vi "Initialise.vi"(8 "error in (no error)":errorcluster, 10 "Window Height":i32=480, 11 "Window Width":i32=640) -> (0 "error out":errorcluster, 3 "Renderer out":refnum<class "Renderer.lvclass">)   [LabVIEW 2021, in "Renderer.lvclass"]
uses:
  Renderer.lvclass
  Renderer.lvclass/Renderer.ctl
  LabSDL2/Source/Libraries/LibSDL2 Wrapper/LibSDL2.lvlib
  LabSDL2/Source/Libraries/LibSDL2_Image Wrapper/LibSDL2_Image.lvlib
  LabSDL2/Source/Libraries/LibSDL2_TTF Wrapper/LibSDL2_TTF.lvlib
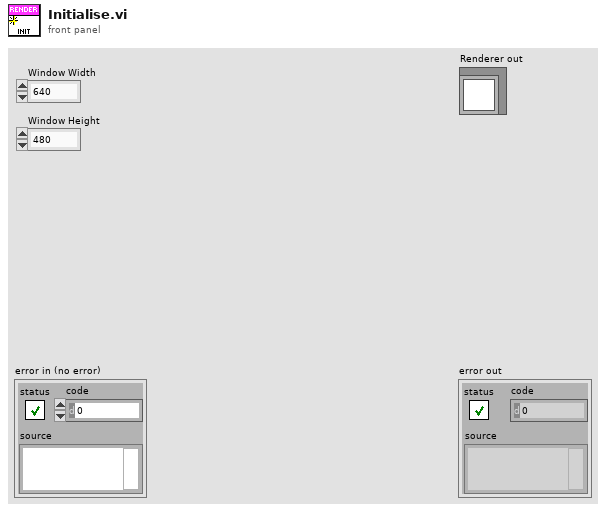
[diagram p1: front panel]
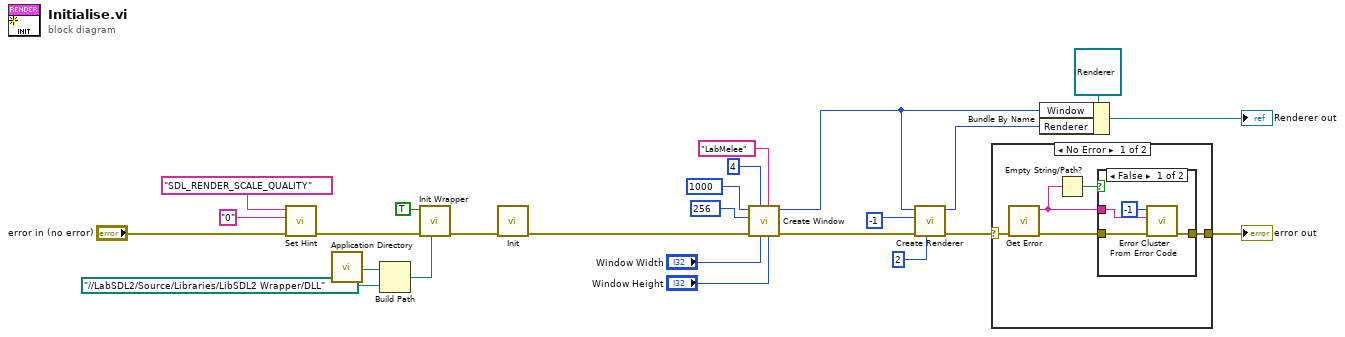
[diagram p0: block diagram]
diagram:
  n1 = call "Set Hint.vi"("error in"="error in (no error)", "Value"="0", "Name"="SDL_RENDER_SCALE_QUALITY") -> ("error out"=w22:errorcluster)  [unwired: 7 in, 1 out]
  n2 = call <vilib>:"Application Directory.vi"() -> ("Application Directory"=w14:path)
  n3 = Build Path(base path=w14, name or relative path=path "../../LabSDL2/Source/Libraries/LibSDL2 Wrapper/DLL" ("DLL Directory")) -> (appended path=w12:path)
  n4 = call "Init Wrapper.vi"("DLL Directory"=w12, "error in"=w22, "PNG (F)"=TRUE ("PNG")) -> ("error out"=w11:errorcluster)  [unwired: 7 in, 1 out]
  n5 = call "Init.vi"("error in (no error)"=w11) -> ("error out"=w10:errorcluster)  [unwired: 9 in, 1 out]
  n6 = call "Create Window.vi"("Height"="Window Height", "Title"="LabMelee", "Width"="Window Width", "Flags"=u32 4, "error in"=w10, "Position y"=u32 256 ("Flags"), "Position x"=u32 1000 ("Flags")) -> ("error out"=w17:errorcluster, "Window Pointer"=w9:u32)  [unwired: 3 in]
  n7 = call "Create Renderer.vi"("Flags"=u32 2, "error in"=w17, "Index"=-1, "Window Pointer"=w9) -> ("error out"=w4:errorcluster, "Renderer Pointer"=w8:u32)  [unwired: 6 in]
  n8 = case shown="No Error" w4 {
    selector: w4 -> [w30 w36]
    tunnel: [w27 w36] -> w3
    frame No Error {
      n9 = call "Get Error.vi"("error in"=w30) -> ("error out"=w28:errorcluster, "Error"=w26:string)  [unwired: 9 in]
      n10 = Empty String/Path?(string/path=w26) -> (empty?=w29:bool)
      n11 = case shown="False" w29 {
        tunnel: w28 -> [w34 w35]
        tunnel: [w31 w35] -> w27
        tunnel: w26 -> [w32 _]
        frame False {
          n12 = call <vilib>:"Error Cluster From Error Code.vi"("error in (no error)"=w34, "error message (\"\")"=w32, "error code (0)"=-1) -> ("error out"=w31:errorcluster)  [unwired: 6 in]
        }
        frame True {
        }
      }
    }
    frame Error {
    }
  }
  "error out" <- w3
  n13 = Bundle By Name(cluster=refnum<class "Renderer.lvclass"> refnum ("Renderer in"), "Window"=w9, "Renderer"=w8) -> (→"Renderer out":refnum<class "Renderer.lvclass">)
